vi "Insert.vi"(6 "commandTimeout":i32, 7 "SqlMapper in":refnum<class "SqlMapper.lvclass">=refnum, 8 "error in (no error)":errorcluster, 9 "DynamicParameters":refnum<class "DynamicParameters.lvclass">=refnum, 10 "tableName":string, 11 "KDBConnection in":refnum<class "KDBConnection.lvclass">=refnum) -> (0 "error out":errorcluster, 2 "id":variant, 3 "KDBConnection out":refnum<class "KDBConnection.lvclass">, 5 "SqlMapper out":refnum<class "SqlMapper.lvclass">)   [LabVIEW 2020]
uses:
  Dapper/SqlMapper/SqlMapper.lvclass
  KDBConnection.lvclass
  Dapper/DynamicParameters/DynamicParameters.lvclass
panel:
  out "affectedRows":i32
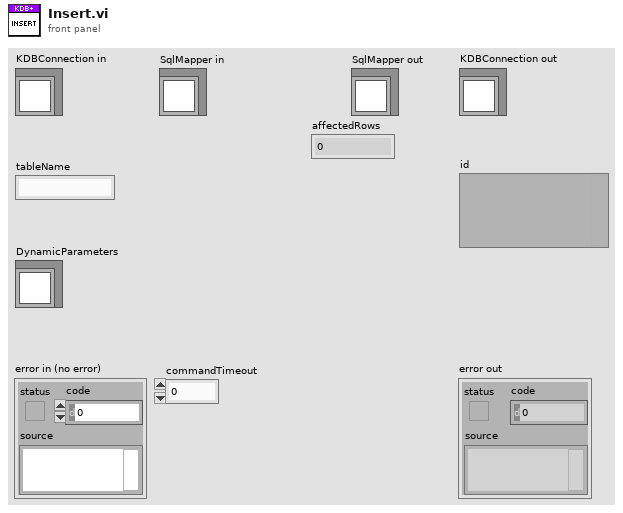
[diagram p1: front panel]
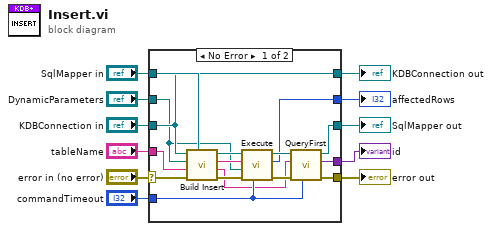
[diagram p0: block diagram]
diagram:
  n1 = case shown="No Error" "error in (no error)" {
    selector: "error in (no error)" -> [w24 w29]
    tunnel: [w21 w29] -> w2
    tunnel: [w16 w28] -> w5
    tunnel: "KDBConnection in" -> [w16 w28]
    tunnel: "SqlMapper in" -> [w26 w27]
    tunnel: "DynamicParameters" -> [w12 _]
    tunnel: [w17 _] -> w3
    tunnel: "commandTimeout" -> [w20 _]
    tunnel: [w18 w27] -> w4
    tunnel: "tableName" -> [w13 _]
    tunnel: [w15 _] -> w1
    frame No Error {
      n2 = call-dynamic "Build Insert.vi"("error in (no error)"=w24, "tableName"=w13, "DynamicParameters in"=w12, "KDBConnection in"=w16) -> ("error out"=w25:errorcluster, "LastIdentityQuery"=w14:string, "InsertStatement"=w23:string)  [unwired: 5 in]
      n3 = call-dynamic "Execute.vi"("commandTimeout"=w20, "error in (no error)"=w25, "DynamicParameters"=w12, "sql"=w23, "SqlMapper in"=w26) -> ("error out"=w22:errorcluster, "affectedRows"=w15:i32, "SqlMapper out"=w19:refnum<class "SqlMapper.lvclass">)  [unwired: 4 in]
      n4 = call-dynamic "QueryFirst.vi"("commandTimeout in"=w20, "error in (no error)"=w22, "sql"=w14, "SqlMapper in"=w19) -> ("error out"=w21:errorcluster, "Value"=w17:variant, "SqlMapper out"=w18:refnum<class "SqlMapper.lvclass">)  [unwired: 5 in]
    }
    frame Error {
    }
  }
  "error out" <- w2
  "KDBConnection out" <- w5
  "id" <- w3
  "SqlMapper out" <- w4
  "affectedRows" <- w1
